vi "Write Most Recent Data Points.vi"(8 "error in (no error)":errorcluster, 10 "Data Points":T1, 11 "Readable in":refnum<class "Readable.lvclass">) -> (0 "error out":errorcluster, 3 "Readable out":refnum<class "Readable.lvclass">)   [LabVIEW 2012, in "Readable.lvclass"]
uses:
  Readable.lvclass
  Data Points.ctl
  Data Point.ctl
  Time.ctl
  X.ctl
  Readable.lvclass/Readable.ctl
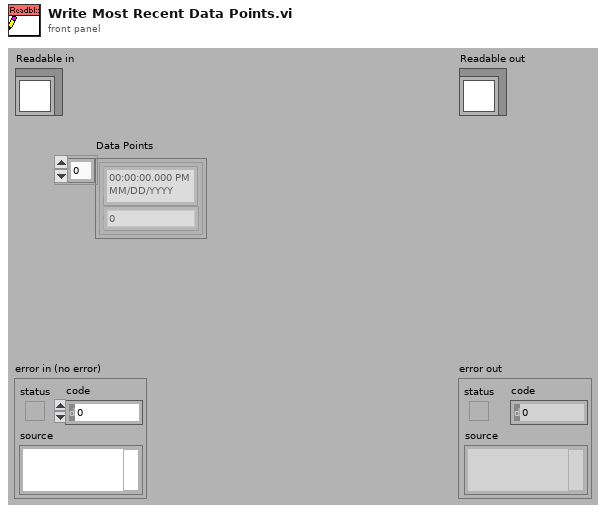
[diagram p1: front panel]
types:
  T1 = typedef "Readable.lvclass/Data Points.ctl" = T2[]
  T2 = typedef "Readable.lvclass/Data Point.ctl" = cluster{"t":T3, "x":T4}
  T3 = typedef "Readable.lvclass/Time.ctl" = timestamp
  T4 = typedef "Readable.lvclass/X.ctl" = dbl
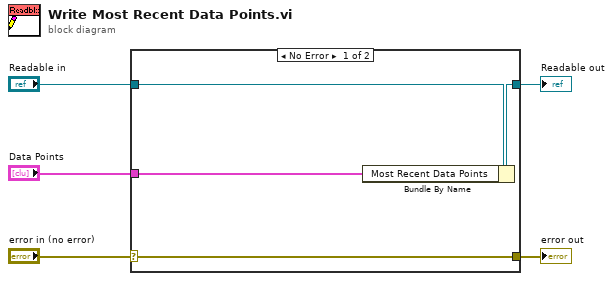
[diagram p0: block diagram]
diagram:
  n1 = case shown="No Error" "error in (no error)" {
    selector: "error in (no error)" -> [w9 w10]
    tunnel: [w9 w10] -> w4
    tunnel: [w7 w11] -> w2
    tunnel: "Readable in" -> [w8 w11]
    tunnel: "Data Points" -> [w6 _]
    frame No Error {
      n2 = Bundle By Name(cluster=w8, "Most Recent Data Points"=w6) -> (w7:refnum<class "Readable.lvclass">)
    }
    frame Error {
    }
  }
  "error out" <- w4
  "Readable out" <- w2
